vi "Global Varibles.vi"() -> ()   [LabVIEW 2023]
panel:
  out "Remaining Time":dbl
  out "Elapsed Time":dbl
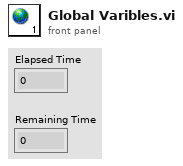
[diagram p1: front panel]
diagram:
